vi "Control Panel.vi"(8 "error in (no error)":errorcluster, 11 "Fake CCD in":refnum<class "Synapse CCD.lvclass">) -> (0 "error out":errorcluster, 3 "Fake CCD out":refnum<class "Synapse CCD.lvclass">)   [LabVIEW 2017, in "Synapse CCD.lvclass"]
doc: "(Dynamic) A user-level application that simulates the physical front panel of the Instrument. Provide the user with buttons to manually control features of the instrument, and provide indicators of its current state."
uses:
  Synapse CCD.lvclass
  Areas.ctl
  <vilib>/Utility/error.llb/DialogType.ctl
  Synapse CCD.lvclass/Synapse CCD.ctl
  Spectrometer Triax 550/JY-SPEX-TRIAX/controls.llb/Slits.ctl
  Global/GPIB Numbers.vi
  Spectrometer Triax 550/JY-SPEX-TRIAX/JY-SPEX-TRIAX.lvlib
  Utility Classes/Readable/Readable.lvclass
panel:
  in  "trigger Set CCD warning":bool=TRUE
  out "Changed setting hit Set CCD before continuing":bool
  out "Status":string
  out "Max slit resolution":dbl[unit]
  out "Warning: counts \nwent too high!":bool
  in  "Go to start\nof raster scan":bool
  out "Current snapshot":i32
  out "Number of data \npoints required":i32
  out "JYCCDLib.IJYCCDReqd 1":refnum<k7>
  out "new version of 2D Emma and John Array":i32[][](array[numeric])
  out "where am i?":string
  out "populate fields with member data: CCD private data":T2={"JYCCDLib.IJYCCDReqd"=refnum, "JYMONOLib.IJYMonoReqd"=refnum, "Integration time"=0.01, "ADC"=0, "GAIN"=0, "Areas"=[[1, 1, 1, 1024, 256, 1, 256]], "Most Recent Data Object"=refnum, "Mono Properties"={"Grating"=0, "Center Wavelength"=0.0, "Entrance Slit"=0.0, "Exit Slit"=0.0}, "Coverage"={"Max"=0.0, "Min"=0.0}, "Multi-Acquisitions"={"Dark Subtract?"=FALSE, "Averaging?"=FALSE, "Cosmic Ray Removal?"=FALSE, "# to Average"=0, "Time Between Acq."=0, "Acquisitions Control Array"=[TRUE], "Raw Data"=[], "Processed Data"=[], "Array of Wavelengths"=[]}, "Raster Scan"={"Raster Scan?"=FALSE, "Start"=0.0, "End"=0.0, "Bin width (pixels)"=1, "Bin width (nm)\n(scan resolution)"=3.7e-11, "Number of CCD bins to use each snapshot"=1, "Total possible CCD bins"=20.48, "Warning: counts \nwent too high!"=FALSE}} {"Raster Scan"."Number of CCD bins to use each snapshot" min=1 max=1024 step=1; "Raster Scan"."Bin width (pixels)" min=1 max=1024 step=1; "Mono Properties"."Grating" items=["1200 lines/mm - 500 nm Blaze", "1200 lines/mm - 750 nm Blaze", "600 lines/mm - 1000 nm Blaze"]; "GAIN" items=["High Light", "Best Dynamic", "High Sensitivity"]; "ADC" items=["   20 kHz", "1 MHz", "1 MHz Ultra"]}
  out "Number of snap-\nshots required":i32
  out "Expected time":dbl[unit]
  out "Total possible CCD bins":dbl=20.48
  out "Cosmic Ray Locations":string
  in  "Raster explanation":bool
  in  "image mode":bool
  in  "Repeat pause (ms)":u32
  out "Max value of last snapshot":i32
  in  "Number of CCD bins to use each snapshot":i32=1 min=1 max=1024 step=1
  out "Bin width (nm)\n(scan resolution)":dbl[unit]=3.7e-11
  in  "Bin width (pixels)":i32=1 min=1 max=1024 step=1
  in  "Start":dbl[unit]
  in  "End":dbl[unit]
  in  "Raster Scan":bool
  in  "Repeat Capture":bool
  out "CCD \nInitialized":bool
  out "Spectrometer \nInitialized":bool
  out "Resolution\n(nm/pixel)":dbl[unit] format="%#_3g"
  in  "File Name":path
  in  "Comments":string
  in  "Export\nPlot":bool
  in  "Cosmic Ray\nRemoval?":bool
  out "UnProcessed Spectra":T3(graph)
  in  "# to Average":u32=1
  in  "Averaging?":bool
  in  "Time Between Acq. (ms)":u32
  out "Spectrum":cluster{"Ramp Pattern":dbl[], "X array":dbl[]}[](graph)
  in  "Take Spectrum":bool
  in  "Set CCD":bool
  in  "Set Grating":bool
  in  "stop":bool
  in  "Exit Slit":dbl[unit]
  in  "Entrance Slit":dbl[unit]
  out "Min":dbl[unit]
  out "Max":dbl[unit]
  in  "Center Wavelength":dbl[unit]
  in  "Grating":u16(ring) items=["1200 lines/mm - 500 nm Blaze", "1200 lines/mm - 750 nm Blaze", "600 lines/mm - 1000 nm Blaze"]
  in  "GAIN":u16(ring) caption="Device Name" items=["High Light", "Best Dynamic", "High Sensitivity"]
  in  "ADC":u16(ring) caption="Device Name" items=["   20 kHz", "1 MHz", "1 MHz Ultra"]
  in  "Integration time":dbl[unit]=0.01
  in  "Dark Subtract?":bool
  in  "Copy Actual to Set":bool
  in  "Populate Fields with Member Data":bool
  # "Running this program automatically moves mirror to CCD position"
  # "(unselect to interrupt scan)"
  # "(keep below 65,536 or it saturates)"
  # "Number of CCD bins used in a snapshot must be smaller than Total possible CCD bins"
  # "Debugging stuff"
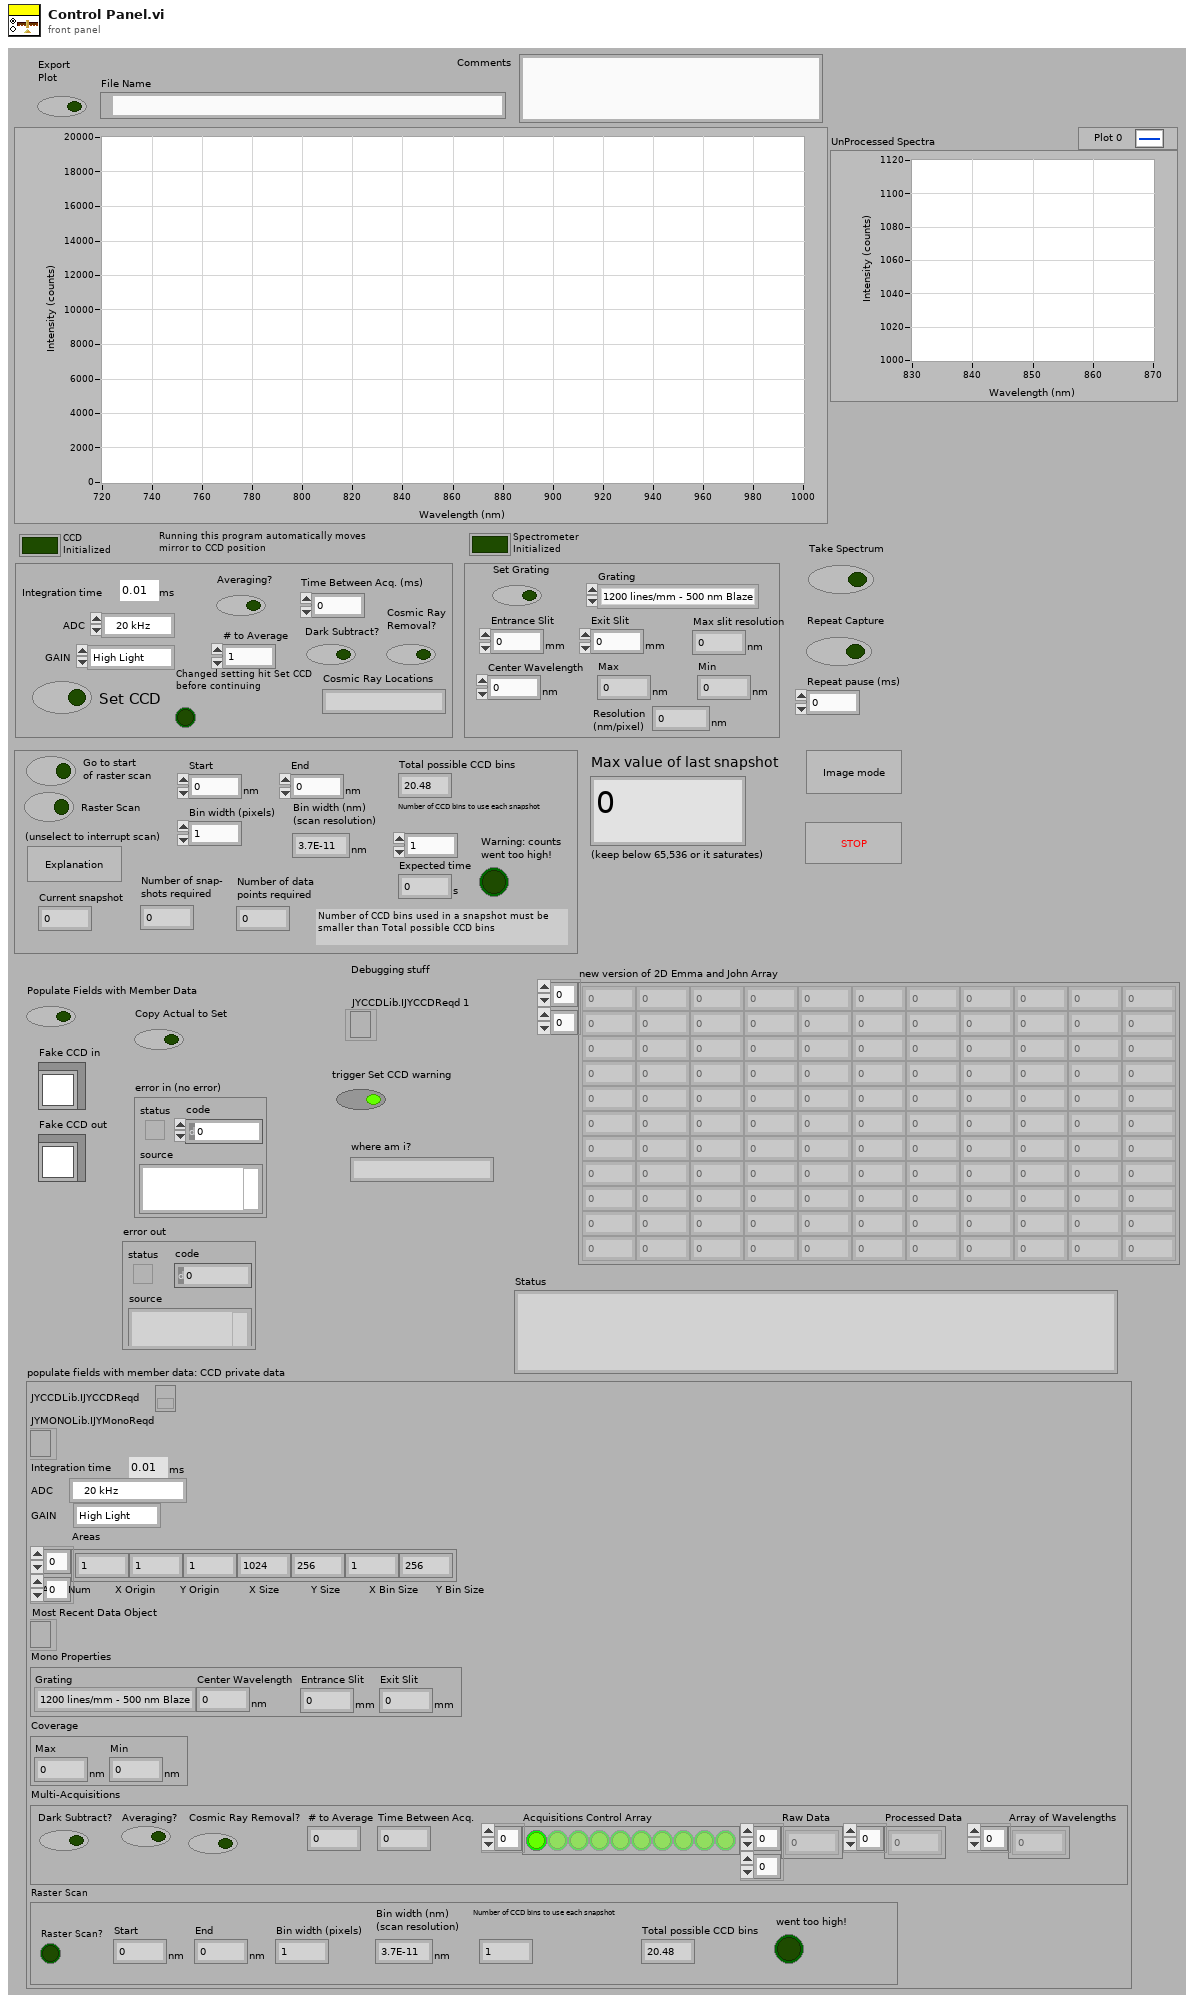
[diagram p1: front panel]
types:
  T1 = typedef "Synapse CCD.lvclass/Areas.ctl" = i32[][]
  T2 = cluster{"JYCCDLib.IJYCCDReqd":refnum<k7>, "JYMONOLib.IJYMonoReqd":refnum<k7>, "Integration time":dbl[unit], "ADC":u16, "GAIN":u16, "Areas":T1, "Most Recent Data Object":refnum<k7>, "Mono Properties":cluster{"Grating":u16, "Center Wavelength":dbl[unit], "Entrance Slit":dbl[unit], "Exit Slit":dbl[unit]}, "Coverage":cluster{"Max":dbl[unit], "Min":dbl[unit]}, "Multi-Acquisitions":cluster{"Dark Subtract?":bool, "Averaging?":bool, "Cosmic Ray Removal?":bool, "# to Average":u32, "Time Between Acq.":u32, "Acquisitions Control Array":bool[], "Raw Data":i32[][], "Processed Data":dbl[], "Array of Wavelengths":dbl[]}, "Raster Scan":cluster{"Raster Scan?":bool, "Start":dbl[unit], "End":dbl[unit], "Bin width (pixels)":i32, "Bin width (nm)\n(scan resolution)":dbl[unit], "Number of CCD bins to use each snapshot":i32, "Total possible CCD bins":dbl, "Warning: counts \nwent too high!":bool}}
  T3 = cluster{"Array of Wavelengths":dbl[], "Raw Data":i32[]}[]
  T4 = typedef "DialogType.ctl" = u16
  T5 = typedef "GPIB Type Def.ctl" = cluster{"Name":string, "bus":dbl, "GPIB":dbl, "GPIB as string":string, "byte":i32, "VISA Resource Name":refnum<visa-resource-name>}
  T6 = typedef "JY-SPEX-TRIAX.lvlib/Slits.ctl" = enum16{"0 (Front/Axial Entrance)", "1 (Side/Lateral Entrance)", "2 (Front/Axial Exit)", "3 (Side/Lateral Exit)"}
  T7 = cluster{"Grating":u16, "Center Wavelength":dbl[unit], "Entrance Slit":dbl[unit], "Exit Slit":dbl[unit]}
  T8 = cluster{"Dark Subtract?":bool, "Averaging?":bool, "Cosmic Ray Removal?":bool, "# to Average":u32, "Time Between Acq.":u32, "Acquisitions Control Array":bool[], "Raw Data":i32[][], "Processed Data":dbl[], "Array of Wavelengths":dbl[]}
  T9 = cluster{"Raster Scan?":bool, "Start":dbl[unit], "End":dbl[unit], "Bin width (pixels)":i32, "Bin width (nm)\n(scan resolution)":dbl[unit], "Number of CCD bins to use each snapshot":i32, "Total possible CCD bins":dbl, "Warning: counts \nwent too high!":bool}
  T10 = cluster{"Array of Wavelengths":dbl[], "Raw Data":i32[]}
  T11 = cluster{"Array of Wavelengths":dbl[], "Processed Data":dbl[]}
  T12 = cluster{"Wavelengths":dbl[], "Avg Counts":dbl[]}[]
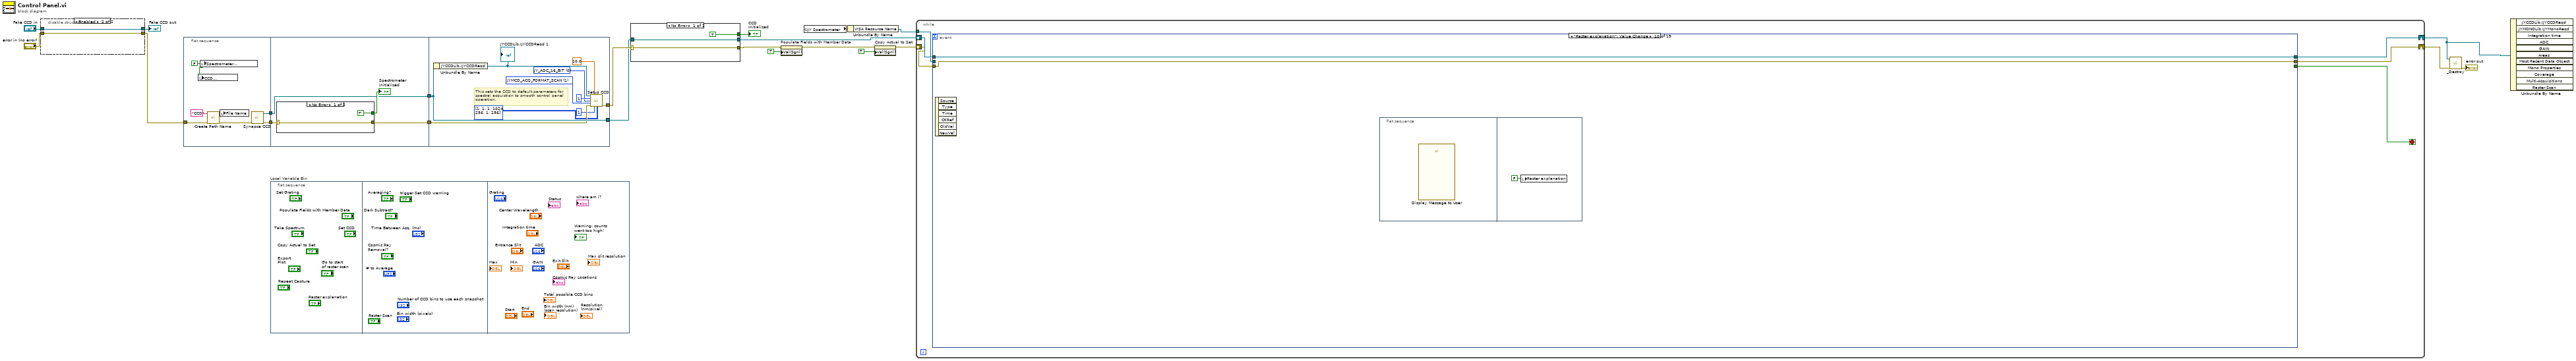
[diagram p0: block diagram]
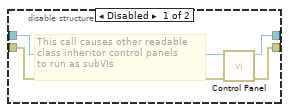
[diagram p2: hidden frame]
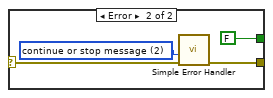
[diagram p3: hidden frame]
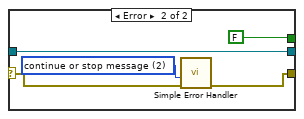
[diagram p4: hidden frame]
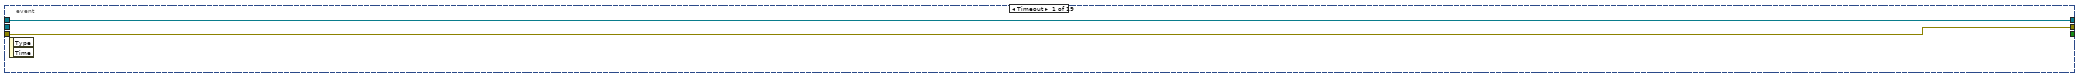
[diagram p5: hidden frame]
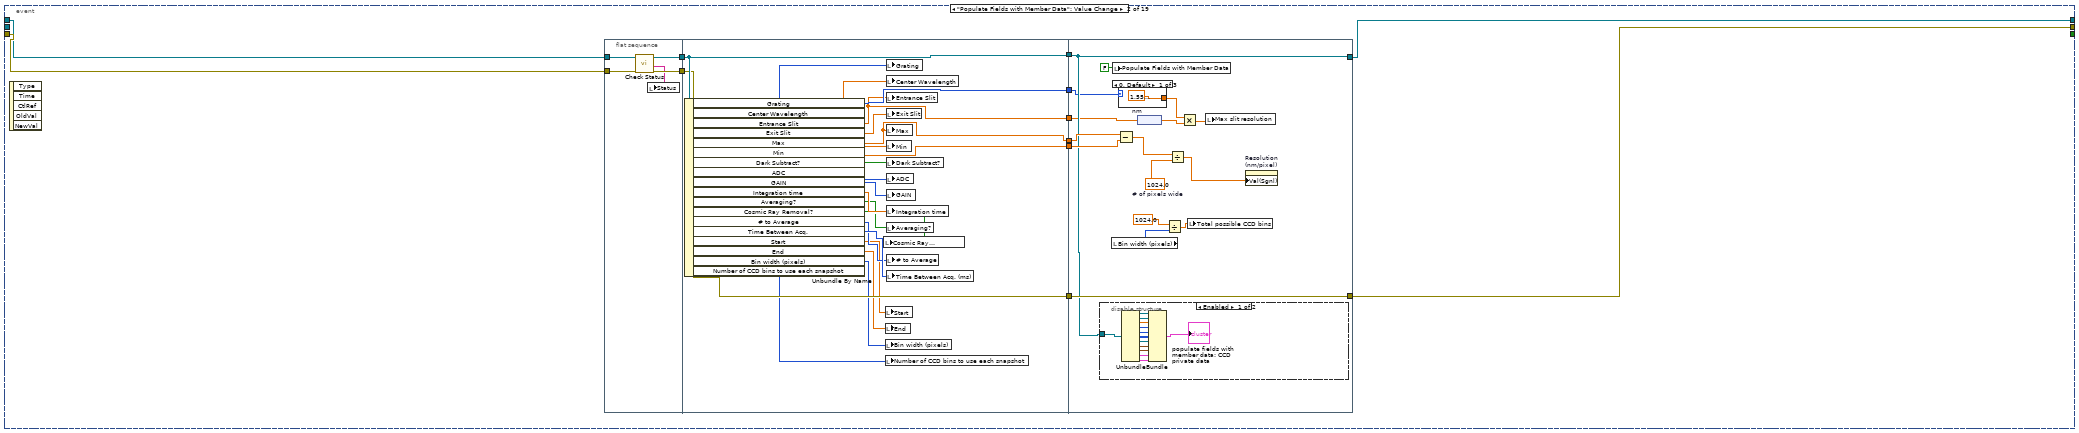
[diagram p6: hidden frame]
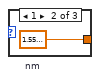
[diagram p7: hidden frame]
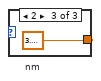
[diagram p8: hidden frame]
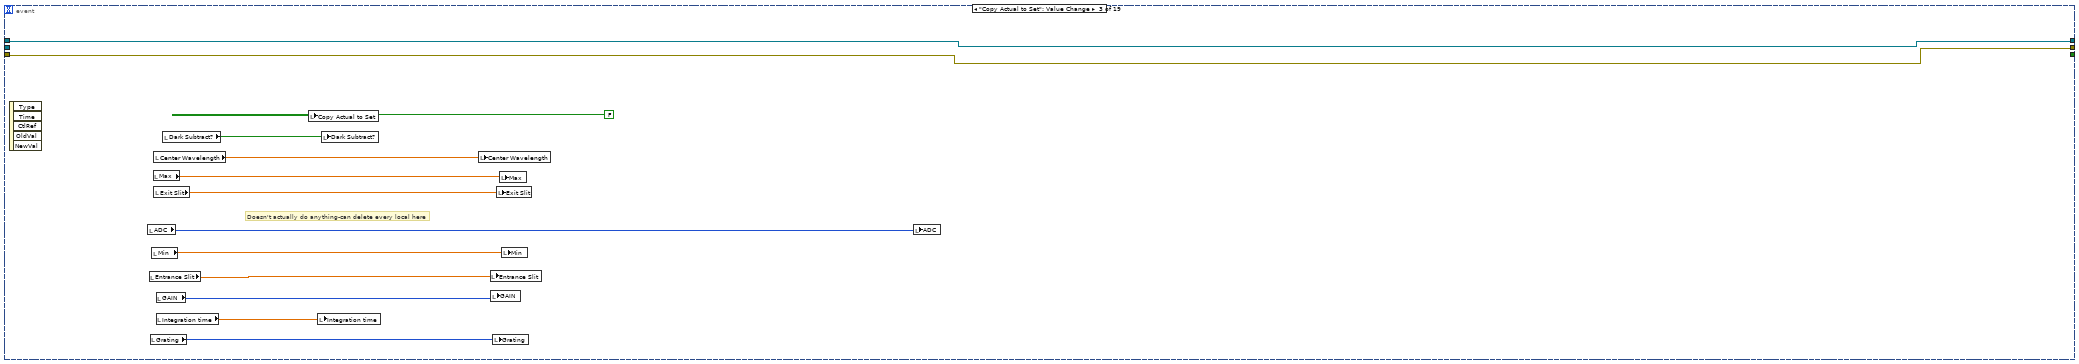
[diagram p10: hidden frame]
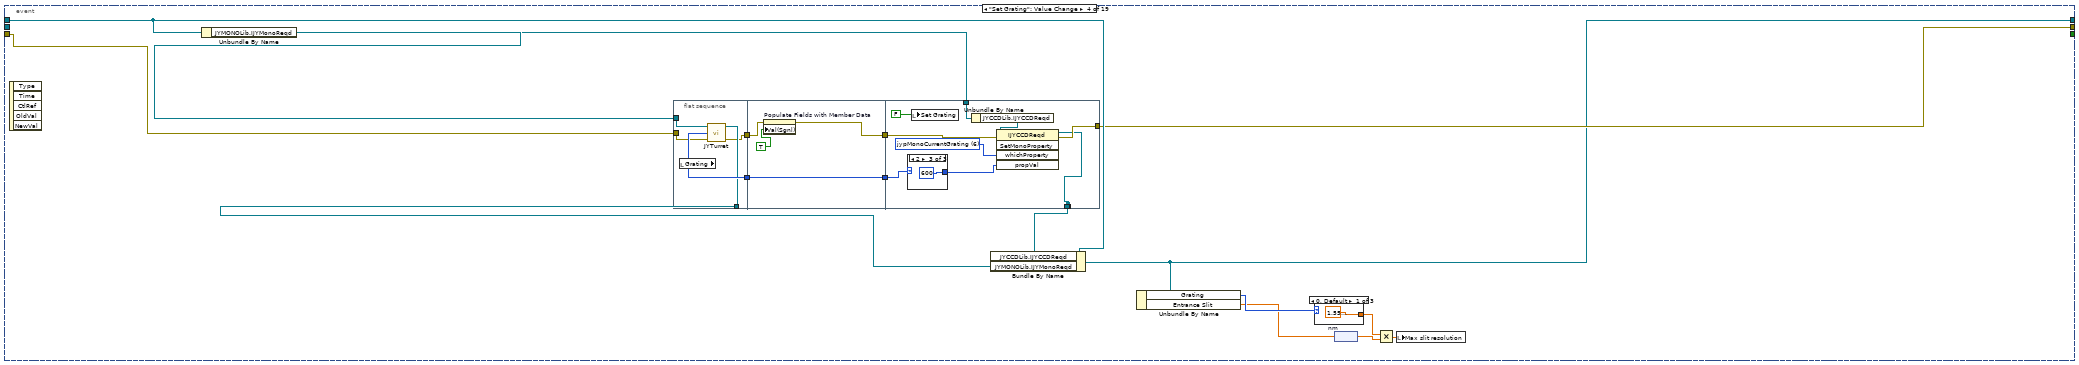
[diagram p11: hidden frame]
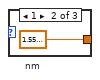
[diagram p12: hidden frame]
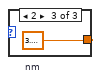
[diagram p13: hidden frame]
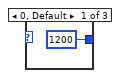
[diagram p14: hidden frame]
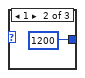
[diagram p15: hidden frame]
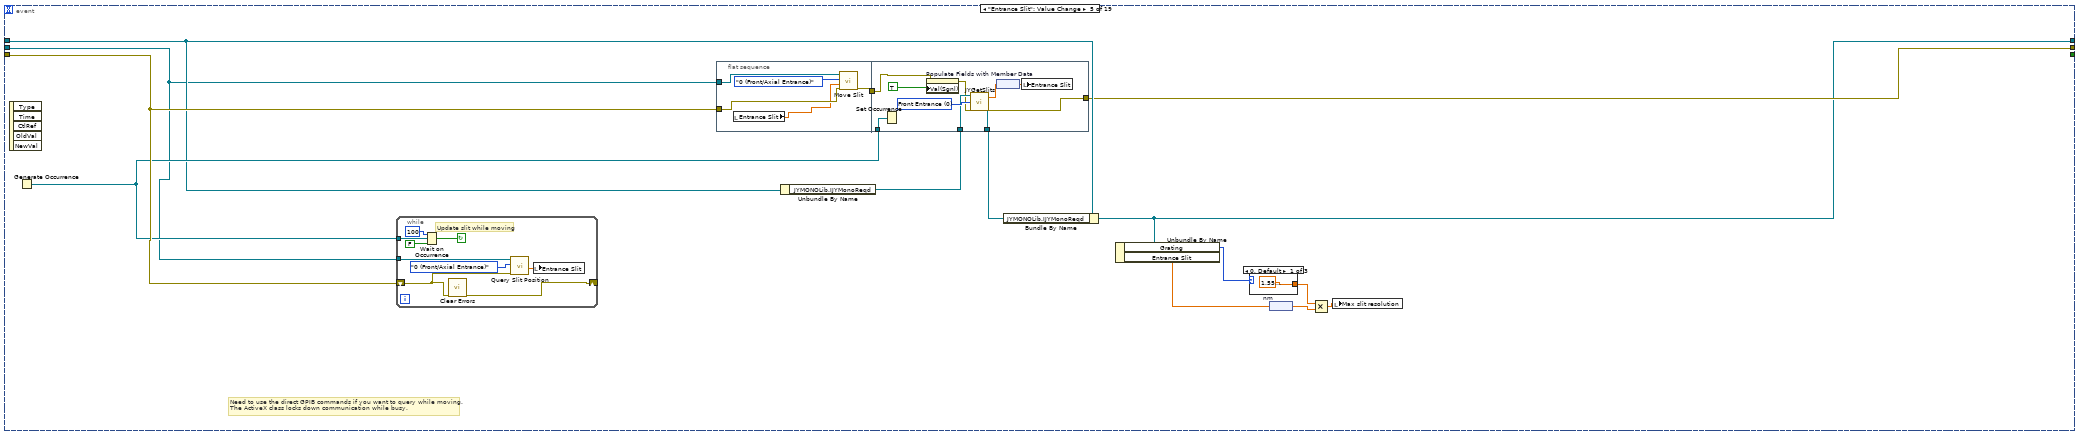
[diagram p16: hidden frame]
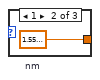
[diagram p17: hidden frame]
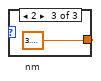
[diagram p18: hidden frame]
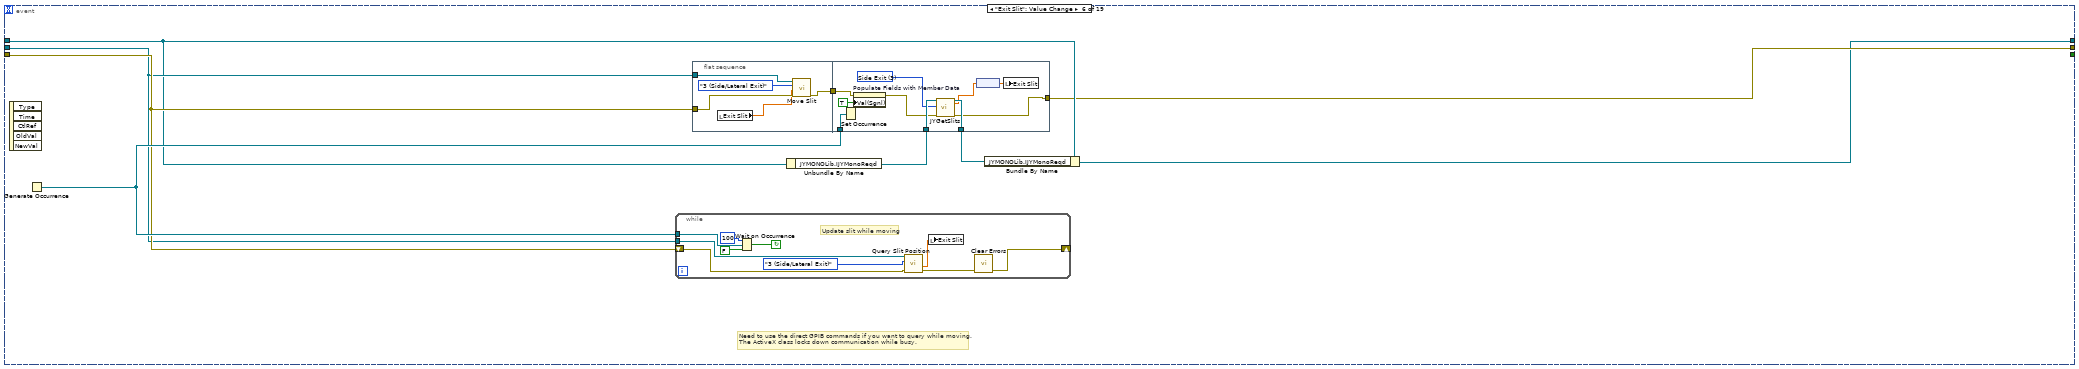
[diagram p19: hidden frame]
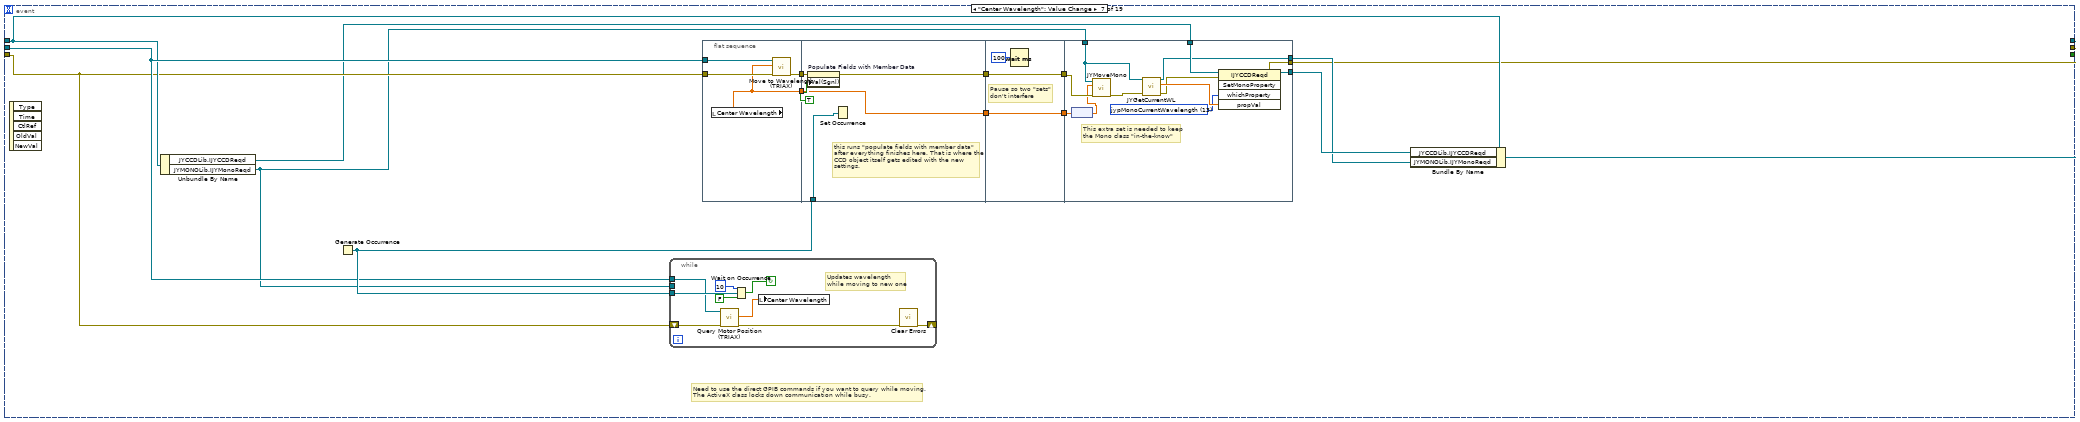
[diagram p20: hidden frame]
diagram:
  n1 = disable-structure shown="Enabled" {
    disable-tunnel: [w26 w28] -> w22
    disable-tunnel: "error in (no error)" -> [w25 w27]
    disable-tunnel: "Fake CCD in" -> [w24 w28]
    disable-tunnel: [w23 w27] -> w19
    frame Disabled {
      # "This call causes other readable\nclass inheritor control panels\nto run as subVIs"
      n2 = call-parent "Control Panel.vi"("error in (no error)"=w25, "Instrument in"=w24) -> ("error out"=w23:errorcluster, "Instrument out"=w26:refnum<class "Synapse CCD.lvclass">)  [unwired: 8 in]
    }
    frame Enabled {
    }
  }
  "Fake CCD out" <- w22
  n3 = flat-sequence {
    tunnel: w19 -> [w33]
    tunnel: [w35] -> w8
    tunnel: [w34] -> w6
    tunnel: w8 -> [w39]
    tunnel: [w38] -> w7
    tunnel: w6 -> [w36]
    tunnel: [w36] -> w5
    tunnel: [w55] -> w2
    tunnel: [w46] -> w13
    tunnel: w7 -> [w49]
    tunnel: w5 -> [w55]
    frame #0 {
      w29 = FALSE ("Spectrometer Initialized")
      n4 = local write "CCD \nInitialized"(w29) -> ()
      n5 = local write "Spectrometer \nInitialized"(w29) -> ()
      n6 = call "Create Path Name.vi"("error in"=w33, "filename"="CCD") -> ("error out"=w32:errorcluster, "path"=w30:path)  [unwired: 1 in, 3 out]
      n7 = local write "File Name"(w30) -> ()
      n8 = call "Synapse CCD.vi"("error in (no error)"=w32) -> ("error out"=w35:errorcluster, "Synapse CCD.lvclass"=w34:refnum<class "Synapse CCD.lvclass">)  [unwired: 9 in]
    }
    frame #1 {
      n9 = case shown="No Error" w39 {
        selector: w39 -> [w41 w44]
        tunnel: [w41 w43] -> w38
        tunnel: [TRUE FALSE] -> w37
        frame No Error {
        }
        frame Error {
          w42 = T4 2 items=["no dialog", "OK message", "continue or stop message", "OK message + warnings", "continue/stop + warnings"] ("type of dialog (OK msg:1)")
          n10 = call <vilib>:"Simple Error Handler.vi"("type of dialog (OK msg:1)"=w42, "error in (no error)"=w44) -> ("error out"=w43:errorcluster)  [unwired: 3 in, 4 out]
        }
      }
      "Spectrometer \nInitialized" <- w37
    }
    frame #2 {
      w50 = 1 items=["JYMCD_ACQ_FORMAT_IMAGE", "JYMCD_ACQ_FORMAT_SCAN"] ("Acquisition type")
      w52 = 0 items=["JY_ADC_16_BIT", "JY_ADC_14_BIT", "JY_ADC_18_BIT"] ("Select ADC")
      # "This sets the CCD to default parameters for\nspectral acquistion to smooth control panel\noperation."
      n11 = Unbundle By Name(w55) -> ("JYCCDLib.IJYCCDReqd"=w54:refnum<k7>)
      "JYCCDLib.IJYCCDReqd 1" <- w54
      n12 = call "Setup CCD.vi"("IJYCCDReqd In"=w54, "Integration time(ms)"=10.0 ("IntegrationTime"), "Select ADC"=w52, "Gain"=1, "Acquisition type"=w50, "error in (no error)"=w49, "numAreas"=1, "areas :"=T1 [[1, 1, 1, 1024, 256, 1, 256]] ("Areas")) -> ("error out"=w46:errorcluster)  [unwired: 5 in, 2 out]
    }
  }
  n13 = flat-sequence "Local Variable Bin" {
    frame #0 {
    }
    frame #1 {
    }
    frame #2 {
    }
  }
  n14 = case shown="No Error" w13 {
    selector: w13 -> [w57 w62]
    tunnel: w2 -> [w58 w63]
    tunnel: [w58 w63] -> w12
    tunnel: [w57 w61] -> w11
    tunnel: [TRUE FALSE] -> w4
    frame No Error {
    }
    frame Error {
      w60 = T4 2 items=["no dialog", "OK message", "continue or stop message", "OK message + warnings", "continue/stop + warnings"] ("type of dialog (OK msg:1)")
      n15 = call <vilib>:"Simple Error Handler.vi"("type of dialog (OK msg:1)"=w60, "error in (no error)"=w62) -> ("error out"=w61:errorcluster)  [unwired: 3 in, 4 out]
    }
  }
  "CCD \nInitialized" <- w4
  n16 = property on="Populate Fields with Member Data" class="Bool (strict)"(error in=w11, "Val(Sgnl)"=TRUE ("Value (Signaling)")) -> (error out=w18:errorcluster)  [unwired: 1 in, 1 out]
  n17 = global read "GPIB Numbers.vi" "JY Spectrometer"() -> (w10:T5)
  n18 = Unbundle By Name(w10) -> ("VISA Resource Name"=w9:refnum<visa-resource-name>)
  n19 = property on="Copy Actual to Set" class="Bool (strict)"(error in=w18, "Val(Sgnl)"=TRUE ("Value (Signaling)")) -> (error out=w17:errorcluster)  [unwired: 1 in, 1 out]
  n20 = while {
    shift-right: [w64] -> w3
    shift-left: w17 -> [w68]
    shift-right: [w65] -> w1
    shift-left: w12 -> [w69]
    tunnel: w9 -> [w67]
    stop <- w66 stop-if-true
    n21 = event shown="[9] \"Raster explanation\": Value Change" {
      selector: _ -> [_ _ _ _ _ _ _ _ _ _ _ _ _ _ _ _ _ _ _]
      dyn-events: _ -> [_ _ _ _ _ _ _ _ _ _ _ _ _ _ _ _ _ _ _]
      timeout: _ -> [_ _ _ _ _ _ _ _ _ _ _ _ _ _ _ _ _ _ _]
      tunnel: w69 -> [w71 w76 w142 w163 w203 w237 w281 w323 w366 w369 w376 w413 w558 w563 w608 w658 _ w724 w741]
      tunnel: w68 -> [w70 w83 w141 w165 w206 w241 w273 w331 w365 w368 w377 w414 w557 w564 w609 w661 _ w723 w742]
      tunnel: [w70 w74 w141 w160 w200 w236 w272 w322 w365 w368 w371 w409 w557 w564 w609 w653 _ w721 w742] -> w64
      tunnel: [w71 w75 w142 w157 w197 w235 w271 w321 w366 w369 w380 w410 w558 w562 w607 w659 _ w722 w741] -> w65
      tunnel: [_ _ _ _ _ _ _ _ _ _ _ _ _ _ _ _ _ _ "stop"] -> w66
      tunnel: w67 -> [_ _ _ _ w202 w239 w282 _ _ _ _ w412 _ _ _ _ _ _ _]
      event Timeout {
        n22 = event-data() -> ()  [unwired: 1 in, 2 out]
      }
      event "Populate Fields with Member Data": Value Change {
        n23 = event-data() -> ()  [unwired: 1 in, 5 out]
        n24 = flat-sequence {
          tunnel: w83 -> [w86]
          tunnel: w76 -> [w88]
          tunnel: [w87] -> w80
          tunnel: [w85] -> w79
          tunnel: [w102] -> w82
          tunnel: [w95] -> w81
          tunnel: w80 -> [w102]
          tunnel: w79 -> [w95]
          tunnel: [w97] -> w78
          tunnel: [w96] -> w77
          tunnel: [w94] -> w73
          tunnel: [w93] -> w72
          tunnel: [w124] -> w74
          tunnel: [w115] -> w75
          tunnel: w82 -> [w115]
          tunnel: w81 -> [w124]
          tunnel: w78 -> [w119]
          tunnel: w77 -> [w120]
          tunnel: w73 -> [w113]
          tunnel: w72 -> [w110]
          frame #0 {
            n25 = call-dynamic "Check Status.vi"("error in (no error)"=w86, "Synapse CCD in"=w88) -> ("error out"=w85:errorcluster, "Status"=w84:string, "Synapse CCD out"=w87:refnum<class "Synapse CCD.lvclass">)  [unwired: 6 in, 1 out]
            n26 = local write "Status"(w84) -> ()
          }
          frame #1 {
            n27 = Unbundle By Name(w102) -> ("Grating"=w94:u16, "Center Wavelength"=w108:dbl[unit], "Entrance Slit"=w93:dbl[unit], "Exit Slit"=w107:dbl[unit], "Max"=w97:dbl[unit], "Min"=w96:dbl[unit], "Dark Subtract?"=w106:bool, "ADC"=w105:u16, "GAIN"=w104:u16, "Integration time"=w103:dbl[unit], "Averaging?"=w98:bool, "Cosmic Ray Removal?"=w99:bool, "# to Average"=w100:u32, "Time Between Acq."=w101:u32, "Start"=w92:dbl[unit], "End"=w91:dbl[unit], "Bin width (pixels)"=w90:i32, "Number of CCD bins to use each snapshot"=w89:i32)
            n28 = local write "Cosmic Ray\nRemoval?"(w99) -> ()
            n29 = local write "Start"(w92) -> ()
            n30 = local write "End"(w91) -> ()
            n31 = local write "Bin width (pixels)"(w90) -> ()
            n32 = local write "Number of CCD bins to use each snapshot"(w89) -> ()
            n33 = local write "Grating"(w94) -> ()
            n34 = local write "Center Wavelength"(w108) -> ()
            n35 = local write "Entrance Slit"(w93) -> ()
            n36 = local write "Exit Slit"(w107) -> ()
            n37 = local write "Max"(w97) -> ()
            n38 = local write "Min"(w96) -> ()
            n39 = local write "Dark Subtract?"(w106) -> ()
            n40 = local write "ADC"(w105) -> ()
            n41 = local write "GAIN"(w104) -> ()
            n42 = local write "Integration time"(w103) -> ()
            n43 = local write "Averaging?"(w98) -> ()
            n44 = local write "# to Average"(w100) -> ()
            n45 = local write "Time Between Acq. (ms)"(w101) -> ()
          }
          frame #2 {
            w121 = 1024.0  # # of pixels wide
            n46 = disable-structure shown="Enabled" {
              disable-tunnel: w115 -> [w132 _]
              frame Enabled {
                n47 = Unbundle(w132) -> (w140:refnum<k7>, w139:refnum<k7>, w138:dbl[unit], w137:u16, w136:u16, w135:T1, w134:refnum<k7>, w133:T7, w131:cluster{"Max":dbl[unit], "Min":dbl[unit]}, w130:T8, w129:T9)
                n48 = Bundle("JYCCDLib.IJYCCDReqd"=w140, "JYMONOLib.IJYMonoReqd"=w139, "Integration time"=w138, "ADC"=w137, "GAIN"=w136, "Areas"=w135, "Most Recent Data Object"=w134, "Mono Properties"=w133, "Coverage"=w131, "Multi-Acquisitions"=w130, "Raster Scan"=w129) -> (→"populate fields with member data: CCD private data":T2)  [unwired: 1 in]
              }
              frame Disabled {
              }
            }
            n49 = local read "Bin width (pixels)"() -> (w117:i32)
            n50 = local write "Populate Fields with Member Data"(FALSE ("Populate Fields with Member Data")) -> ()
            n51 = Subtract(x=w119, y=w120) -> (x-y=w122:dbl[unit])
            n52 = case shown="0, Default" w113 {
              tunnel: [w125 w126 w127] -> w112
              frame 0, Default {
                w125 = dbl[unit] 1.5500000000000002e-09  # nm
              }
              frame 1 {
                w126 = dbl[unit] 1.5500000000000002e-09  # nm
              }
              frame 2 {
                w127 = dbl[unit] 3.1000000000000005e-09  # nm
              }
            }
            n53 = node(w110) -> (w109:dbl)
            n54 = Divide(x=1024.0, y=w117) -> (x/y=w118:dbl)
            n55 = Divide(x=w122, y=w121) -> (x/y=w114:dbl[unit])
            n56 = Multiply(x=w112, y=w109) -> (x*y=w111:dbl[unit])
            n57 = local write "Total possible CCD bins"(w118) -> ()
            n58 = local write "Max slit resolution"(w111) -> ()
            n59 = property on="Resolution\n(nm/pixel)" class="DigNum (strict)"("Val(Sgnl)"=w114) -> ()  [unwired: 2 in, 2 out]
          }
        }
      }
      event "Copy Actual to Set": Value Change {
        # "Doesn't actually do anything-can delete every local here"
        n60 = event-data() -> ()  [unwired: 1 in, 5 out]
        n61 = local read "ADC"() -> (w153:u16)
        n62 = local read "Entrance Slit"() -> (w149:dbl[unit])
        n63 = local read "Grating"() -> (w146:u16)
        n64 = local read "Min"() -> (w150:dbl[unit])
        n65 = local read "Max"() -> (w144:dbl[unit])
        n66 = local read "Center Wavelength"() -> (w152:dbl[unit])
        n67 = local read "Exit Slit"() -> (w148:dbl[unit])
        n68 = local read "GAIN"() -> (w147:u16)
        n69 = local read "Integration time"() -> (w145:dbl[unit])
        n70 = local read "Dark Subtract?"() -> (w151:bool)
        n71 = local write "Copy Actual to Set"(FALSE ("Copy Actual to Set")) -> ()
        n72 = local write "Integration time"(w145) -> ()
        n73 = local write "Dark Subtract?"(w151) -> ()
        n74 = local write "Center Wavelength"(w152) -> ()
        n75 = local write "Entrance Slit"(w149) -> ()
        n76 = local write "GAIN"(w147) -> ()
        n77 = local write "Grating"(w146) -> ()
        n78 = local write "Exit Slit"(w148) -> ()
        n79 = local write "Max"(w144) -> ()
        n80 = local write "Min"(w150) -> ()
        n81 = local write "ADC"(w153) -> ()
      }
      event "Set Grating": Value Change {
        n82 = event-data() -> ()  [unwired: 1 in, 5 out]
        n83 = Unbundle By Name(w163) -> ("JYMONOLib.IJYMonoReqd"=w164:refnum<k7>)
        n84 = flat-sequence {
          tunnel: w164 -> [w175]
          tunnel: w165 -> [w176]
          tunnel: [w173] -> w169
          tunnel: [w177] -> w167
          tunnel: [w174] -> w162
          tunnel: w169 -> [w181]
          tunnel: [w180] -> w168
          tunnel: w167 -> [w180]
          tunnel: [w178] -> w166
          tunnel: [w183] -> w160
          tunnel: w168 -> [w189]
          tunnel: w166 -> [w186]
          tunnel: [w182] -> _
          tunnel: w163 -> [w188]
          tunnel: [w182] -> w161
          frame #0 {
            n85 = local read "Grating"() -> (w177:u16)
            n86 = call "JYTurret.vi"("error in (no error)"=w176, "Grating Index"=w177, "JYMONOLib.IJYMonoReqd In"=w175) -> ("error out"=w173:errorcluster, "JYMONOLib.IJYMonoReqd Out"=w174:refnum<k7>)  [unwired: 1 out]
          }
          frame #1 {
            n87 = property on="Populate Fields with Member Data" class="Bool (strict)"(error in=w181, "Val(Sgnl)"=TRUE ("Value (Signaling)")) -> (error out=w178:errorcluster)  [unwired: 1 in, 1 out]
          }
          frame #2 {
            w187 = 6 items=["jyUndefined", "jypMonoLinearDispersion", "jypMonoBacklashAmount", "jypMonoStepsPerUnit", "jypMonoBaseUnits", "jypMonoBaseGrating", "jypMonoCurrentGrating", "jypMonoMaxLimit", "jypMonoMinLimit", "jypMonoTiltAngle", "jypMonoIncludedAngle", "jypMonoFocalLength", "jypMonoOrder", "jypMonoCurrentWavelength", "jypMonoMCDWavelengthDirection", "jypBandpassUnits", "jypSlitMaxLimit", "jypSlitMinLimit", "jypSlitBackLashAmount", "jypSlitBaseUnits", "jypSlitStepsPerUnit", "jypLaserLine", "jypTotalHardwarePropertiesPlusOne", "jypCurrentTurretPosition"] ("whichProperty")
            n88 = case shown="2" w189 {
              tunnel: [u16 1200 u16 1200 u16 600] -> w184
              frame 0, Default {
              }
              frame 1 {
              }
              frame 2 {
              }
            }
            n89 = local write "Set Grating"(FALSE ("Set Spectrometer")) -> ()
            n90 = Unbundle By Name(w188) -> ("JYCCDLib.IJYCCDReqd"=w185:refnum<k7>)
            n91 = invoke class="IJYCCDReqd" method="SetMonoProperty"(reference=w185, error in=w186, "whichProperty"=w187, "propVal"=w184) -> (reference out=w182:refnum<k7>, error out=w183:errorcluster)  [unwired: 1 in, 3 out]
          }
        }
        n92 = Bundle By Name(cluster=w163, "JYCCDLib.IJYCCDReqd"=w161, "JYMONOLib.IJYMonoReqd"=w162) -> (w157:refnum<class "Synapse CCD.lvclass">)
        n93 = Unbundle By Name(w157) -> ("Grating"=w156:u16, "Entrance Slit"=w155:dbl[unit])
        n94 = case shown="0, Default" w156 {
          tunnel: [w170 w171 w172] -> w159
          frame 0, Default {
            w170 = dbl[unit] 1.5500000000000002e-09  # nm
          }
          frame 1 {
            w171 = dbl[unit] 1.5500000000000002e-09  # nm
          }
          frame 2 {
            w172 = dbl[unit] 3.1000000000000005e-09  # nm
          }
        }
        n95 = node(w155) -> (w158:dbl)
        n96 = Multiply(x=w159, y=w158) -> (x*y=w154:dbl[unit])
        n97 = local write "Max slit resolution"(w154) -> ()
      }
      event "Entrance Slit": Value Change {
        # "Need to use the direct GPIB commands if you want to query while moving.\nThe ActiveX class locks down communication while busy."
        n98 = event-data() -> ()  [unwired: 1 in, 5 out]
        n99 = Generate Occurrence() -> (w205:refnum<k4>)
        n100 = while {
          tunnel: w205 -> [w219]
          shift-right: [w211] -> _
          shift-left: w206 -> [w212]
          tunnel: w202 -> [w215]
          stop <- w218 continue-if-true
          # "Update slit while moving"
          n101 = Wait on Occurrence(1:FALSE ("ignore previous (T)"), 2:w219, 3:100 ("ms timeout (-1)")) -> (0:w218:bool)
          n102 = call <vilib>:"Clear Errors.vi"("error in (no error)"=w212) -> ("error out"=w211:errorcluster)  [unwired: 5 in, 1 out]
          n103 = call "Query Slit Position.vi"("error in (no error)"=w212, "Slit (Front/Axial Entrance)"=Slits."0 (Front/Axial Entrance)", "VISA resource name"=w215) -> ("Slit Position"=w213:dbl[unit])  [unwired: 6 in, 2 out]
          n104 = local write "Entrance Slit"(w213) -> ()
        }
        n105 = flat-sequence {
          tunnel: w206 -> [w221]
          tunnel: [w224] -> w207
          tunnel: w202 -> [w222]
          tunnel: w207 -> [w229]
          tunnel: [w225] -> w200
          tunnel: w205 -> [w234]
          tunnel: w204 -> [w232]
          tunnel: [w230] -> w201
          frame #0 {
            n106 = local read "Entrance Slit"() -> (w220:dbl[unit])
            n107 = call "Move Slit.vi"("error in (no error)"=w221, "Desired Slit Position"=w220, "Slit (Front/Axial Entrance)"=Slits."0 (Front/Axial Entrance)", "VISA resource name"=w222) -> ("error out"=w224:errorcluster)  [unwired: 6 in, 1 out]
          }
          frame #1 {
            w233 = u16 0 items=["Front Entrance", "Side Entrance", "Front Exit", "Side Exit", "First Intermediate", "Second Intermediate"] ("Slit")
            n108 = Set Occurrence(w234) -> ()
            n109 = property on="Populate Fields with Member Data" class="Bool (strict)"(error in=w229, "Val(Sgnl)"=TRUE ("Value (Signaling)")) -> (error out=w227:errorcluster)  [unwired: 1 in, 1 out]
            n110 = call "JYGetSlits.vi"("MonoRefNum IN"=w232, "Slit"=w233, "error in (no error)"=w227) -> ("MonoRefNum Out"=w230:refnum<k7>, "Slit Width"=w226:dbl, "error out"=w225:errorcluster)  [unwired: 13 in, 1 out]
            n111 = node(w226) -> (w231:dbl[unit])
            n112 = local write "Entrance Slit"(w231) -> ()
          }
        }
        n113 = Unbundle By Name(w203) -> ("JYMONOLib.IJYMonoReqd"=w204:refnum<k7>)
        n114 = Bundle By Name(cluster=w203, "JYMONOLib.IJYMonoReqd"=w201) -> (w197:refnum<class "Synapse CCD.lvclass">)
        n115 = Unbundle By Name(w197) -> ("Grating"=w196:u16, "Entrance Slit"=w195:dbl[unit])
        n116 = case shown="0, Default" w196 {
          tunnel: [w208 w209 w210] -> w199
          frame 0, Default {
            w208 = dbl[unit] 1.5500000000000002e-09  # nm
          }
          frame 1 {
            w209 = dbl[unit] 1.5500000000000002e-09  # nm
          }
          frame 2 {
            w210 = dbl[unit] 3.1000000000000005e-09  # nm
          }
        }
        n117 = node(w195) -> (w198:dbl)
        n118 = Multiply(x=w199, y=w198) -> (x*y=w194:dbl[unit])
        n119 = local write "Max slit resolution"(w194) -> ()
      }
      event "Exit Slit": Value Change {
        # "Need to use the direct GPIB commands if you want to query while moving.\nThe ActiveX class locks down communication while busy."
        n120 = event-data() -> ()  [unwired: 1 in, 5 out]
        n121 = Generate Occurrence() -> (w242:refnum<k4>)
        n122 = while {
          tunnel: w242 -> [w253]
          shift-right: [w244] -> _
          shift-left: w241 -> [w248]
          tunnel: w239 -> [w247]
          stop <- w251 continue-if-true
          # "Update slit while moving"
          n123 = Wait on Occurrence(1:FALSE ("ignore previous (T)"), 2:w253, 3:100 ("ms timeout (-1)")) -> (0:w251:bool)
          n124 = call "Query Slit Position.vi"("error in (no error)"=w248, "Slit (Front/Axial Entrance)"=Slits."3 (Side/Lateral Exit)", "VISA resource name"=w247) -> ("error out"=w245:errorcluster, "Slit Position"=w249:dbl[unit])  [unwired: 6 in, 1 out]
          n125 = local write "Exit Slit"(w249) -> ()
          n126 = call <vilib>:"Clear Errors.vi"("error in (no error)"=w245) -> ("error out"=w244:errorcluster)  [unwired: 5 in, 1 out]
        }
        n127 = flat-sequence {
          tunnel: w241 -> [w257]
          tunnel: [w254] -> w243
          tunnel: w239 -> [w256]
          tunnel: w243 -> [w262]
          tunnel: [w259] -> w236
          tunnel: w242 -> [w267]
          tunnel: w240 -> [w266]
          tunnel: [w263] -> w238
          frame #0 {
            n128 = local read "Exit Slit"() -> (w255:dbl[unit])
            n129 = call "Move Slit.vi"("error in (no error)"=w257, "Desired Slit Position"=w255, "Slit (Front/Axial Entrance)"=Slits."3 (Side/Lateral Exit)", "VISA resource name"=w256) -> ("error out"=w254:errorcluster)  [unwired: 6 in, 1 out]
          }
          frame #1 {
            w265 = u16 3 items=["Front Entrance", "Side Entrance", "Front Exit", "Side Exit", "First Intermediate", "Second Intermediate"] ("Slit")
            n130 = Set Occurrence(w267) -> ()
            n131 = property on="Populate Fields with Member Data" class="Bool (strict)"(error in=w262, "Val(Sgnl)"=TRUE ("Value (Signaling)")) -> (error out=w261:errorcluster)  [unwired: 1 in, 1 out]
            n132 = call "JYGetSlits.vi"("MonoRefNum IN"=w266, "Slit"=w265, "error in (no error)"=w261) -> ("MonoRefNum Out"=w263:refnum<k7>, "Slit Width"=w260:dbl, "error out"=w259:errorcluster)  [unwired: 13 in, 1 out]
            n133 = node(w260) -> (w264:dbl[unit])
            n134 = local write "Exit Slit"(w264) -> ()
          }
        }
        n135 = Unbundle By Name(w237) -> ("JYMONOLib.IJYMonoReqd"=w240:refnum<k7>)
        n136 = Bundle By Name(cluster=w237, "JYMONOLib.IJYMonoReqd"=w238) -> (w235:refnum<class "Synapse CCD.lvclass">)
      }
      event "Center Wavelength": Value Change {
        # "Need to use the direct GPIB commands if you want to query while moving.\nThe ActiveX class locks down communication while busy."
        n137 = event-data() -> ()  [unwired: 1 in, 5 out]
        n138 = Unbundle By Name(w281) -> ("JYCCDLib.IJYCCDReqd"=w270:refnum<k7>, "JYMONOLib.IJYMonoReqd"=w269:refnum<k7>)
        n139 = Generate Occurrence() -> (w283:refnum<k4>)
        n140 = while {
          tunnel: w283 -> [w293]
          tunnel: w269 -> [_]
          shift-right: [w289] -> _
          shift-left: w273 -> [w288]
          tunnel: w282 -> [w285]
          stop <- w291 continue-if-true
          # "Updates wavelength\nwhile moving to new one"
          n141 = call "Query Motor Position (TRIAX).vi"("error in (no error)"=w288, "VISA resource name"=w285) -> ("error out"=w287:errorcluster, "wavelength"=w286:dbl[unit])  [unwired: 7 in, 1 out]
          n142 = Wait on Occurrence(1:FALSE ("ignore previous (T)"), 2:w293, 3:10 ("ms timeout (-1)")) -> (0:w291:bool)
          n143 = local write "Center Wavelength"(w286) -> ()
          n144 = call <vilib>:"Clear Errors.vi"("error in (no error)"=w287) -> ("error out"=w289:errorcluster)  [unwired: 5 in, 1 out]
        }
        n145 = flat-sequence {
          tunnel: w273 -> [w297]
          tunnel: [w296] -> w284
          tunnel: w282 -> [w295]
          tunnel: [w294] -> w278
          tunnel: w284 -> [w301]
          tunnel: [w300] -> w277
          tunnel: w283 -> [w298]
          tunnel: [w299] -> w275
          tunnel: w278 -> [w299]
          tunnel: w277 -> [w305]
          tunnel: [w305] -> w276
          tunnel: w275 -> [w304]
          tunnel: [w304] -> w274
          tunnel: [w317] -> w272
          tunnel: w276 -> [w310]
          tunnel: w270 -> [w316]
          tunnel: [w313] -> w280
          tunnel: [w307] -> w279
          tunnel: w274 -> [w311]
          tunnel: w269 -> [w306]
          frame #0 {
            n146 = local read "Center Wavelength"() -> (w294:dbl[unit])
            n147 = call "Move to Wavelength (TRIAX).vi"("error in (no error)"=w297, "Target wavelength"=w294, "VISA resource name"=w295) -> ("error out"=w296:errorcluster)  [unwired: 7 in, 1 out]
          }
          frame #1 {
            # "this runs \"populate fields with member data\" \nafter everything finishes here. That is where the \nCCD object itself gets edited with the new \nsettings."
            n148 = property on="Populate Fields with Member Data" class="Bool (strict)"(error in=w301, "Val(Sgnl)"=TRUE ("Value (Signaling)")) -> (error out=w300:errorcluster)  [unwired: 1 in, 1 out]
            n149 = Set Occurrence(w298) -> ()
          }
          frame #2 {
            # "Pause so two \"sets\" \ndon't interfere"
            n150 = Wait (ms)(milliseconds to wait=u32 100) -> ()  [unwired: 1 out]
          }
          frame #3 {
            w308 = 13 items=["jyUndefined", "jypMonoLinearDispersion", "jypMonoBacklashAmount", "jypMonoStepsPerUnit", "jypMonoBaseUnits", "jypMonoBaseGrating", "jypMonoCurrentGrating", "jypMonoMaxLimit", "jypMonoMinLimit", "jypMonoTiltAngle", "jypMonoIncludedAngle", "jypMonoFocalLength", "jypMonoOrder", "jypMonoCurrentWavelength", "jypMonoMCDWavelengthDirection", "jypBandpassUnits", "jypSlitMaxLimit", "jypSlitMinLimit", "jypSlitBackLashAmount", "jypSlitBaseUnits", "jypSlitStepsPerUnit", "jypLaserLine", "jypTotalHardwarePropertiesPlusOne", "jypCurrentTurretPosition"] ("whichProperty")
            # "This extra set is needed to keep \nthe Mono class \"in-the-know\""
            n151 = node(w311) -> (w309:dbl)
            n152 = call "JYMoveMono.vi"("error in (no error)"=w310, 10:w309, "JYMONOLib.IJYMonoReqd"=w306) -> ("error out"=w312:errorcluster)  [unwired: 8 in]
            n153 = call "JYGetCurrentWL.vi"("error in (no error)"=w312, "JYMONOLib.IJYMonoReqd In"=w306) -> ("error out"=w314:errorcluster, "Current WL"=w315:dbl, "JYMONOLib.IJYMonoReqd Out"=w307:refnum<k7>)  [unwired: 6 in, 1 out]
            n154 = invoke class="IJYCCDReqd" method="SetMonoProperty"(reference=w316, error in=w314, "whichProperty"=w308, "propVal"=w315) -> (reference out=w313:refnum<k7>, error out=w317:errorcluster)  [unwired: 1 in, 3 out]
          }
        }
        n155 = Bundle By Name(cluster=w281, "JYCCDLib.IJYCCDReqd"=w280, "JYMONOLib.IJYMonoReqd"=w279) -> (w271:refnum<class "Synapse CCD.lvclass">)
      }
      event "Set CCD": Value Change {
        # "ADC Query Method is broken\n\nKeep track of it manually in \nmember data"
        n156 = event-data() -> ()  [unwired: 1 in, 5 out]
        n157 = Unbundle By Name(w323) -> ("JYCCDLib.IJYCCDReqd"=w318:refnum<k7>, "Areas"=w326:T1)
        n158 = local write "where am i?"("step1" ("where am i?")) -> ()
        n159 = Index Array(array=w326, index (col)=0 ("index (row)")) -> (element=w325:i32[])  [unwired: 1 in]
        n160 = Array Size(array=w325) -> (size(s)=w324:i32)
        n161 = flat-sequence {
          tunnel: w324 -> [w345]
          tunnel: w326 -> [w344]
          tunnel: w318 -> [w338]
          tunnel: w331 -> [w339]
          tunnel: [w342] -> w330
          tunnel: w323 -> [w341]
          tunnel: [w333] -> w327
          tunnel: w330 -> [w351]
          tunnel: [w351] -> w328
          tunnel: [w347] -> w321
          tunnel: w327 -> [w350]
          tunnel: w328 -> [w358]
          tunnel: [w357] -> w320
          tunnel: [w363] -> w322
          tunnel: w320 -> [w363]
          frame #0 {
            w336 = 1 items=["JYMCD_ACQ_FORMAT_IMAGE", "JYMCD_ACQ_FORMAT_SCAN"] ("Acquisition type")
            n162 = local read "Integration time"() -> (w343:dbl[unit])
            n163 = node(w343) -> (w335:dbl)
            n164 = local read "GAIN"() -> (w337:u16)
            n165 = local read "ADC"() -> (w334:u16)
            n166 = call "Setup CCD.vi"("IJYCCDReqd In"=w338, "Integration time(ms)"=w335, "Select ADC"=w334, "Gain"=w337, "Acquisition type"=w336, "error in (no error)"=w339, "numAreas"=w345, "areas :"=w344) -> ("IJYCCDReqd Out"=w340:refnum<k7>, "error out"=w342:errorcluster)  [unwired: 5 in, 1 out]
            n167 = local write "where am i?"("step2" ("where am i?")) -> ()
            n168 = Bundle By Name(cluster=w341, "ADC"=w334, "JYCCDLib.IJYCCDReqd"=w340) -> (w333:refnum<class "Synapse CCD.lvclass">)
          }
          frame #1 {
            n169 = local read "Time Between Acq. (ms)"() -> (w352:u32)
            n170 = local read "Averaging?"() -> (w349:bool)
            n171 = local read "Cosmic Ray\nRemoval?"() -> (w348:bool)
            n172 = local read "Dark Subtract?"() -> (w354:bool)
            n173 = local read "# to Average"() -> (w353:u32)
            n174 = local write "where am i?"("step3" ("where am i?")) -> ()
            n175 = call "Setup Multi Acq.vi"("# of Scans"=w353, "Time Between Acq (ms)"=w352, "Cosmic Ray Removal?"=w348, "Averaging?"=w349, "Dark Subtract?"=w354, "Synapse CCD.lvclass In"=w350) -> ("Synapse CCD.lvclass Out"=w347:refnum<class "Synapse CCD.lvclass">)  [unwired: 5 in]
          }
          frame #2 {
            n176 = property on="Populate Fields with Member Data" class="Bool (strict)"(error in=w358, "Val(Sgnl)"=TRUE) -> (error out=w357:errorcluster)  [unwired: 1 in, 1 out]
            n177 = local write "where am i?"("step4" ("where am i?")) -> ()
            n178 = Wait (ms)(milliseconds to wait=u32 100) -> ()  [unwired: 1 out]
          }
          frame #3 {
            n179 = local write "where am i?"("step5" ("where am i?")) -> ()
            n180 = local write "Set CCD"(FALSE ("Set CCD")) -> ()
            "Changed setting hit Set CCD before continuing" <- FALSE ("Set CCD")
          }
        }
      }
      event "Cosmic Ray\nRemoval?", "ADC", "GAIN", "Time Between Acq. (ms)", "trigger Set CCD warning": Value Change {
        n181 = event-data() -> ()  [unwired: 1 in, 6 out]
        n182 = local write "Changed setting hit Set CCD before continuing"(TRUE ("trigger Set CCD warning")) -> ()
        n183 = local write "trigger Set CCD warning"(FALSE ("trigger Set CCD warning")) -> ()
      }
      event "Raster explanation": Value Change {
        n184 = event-data() -> ()  [unwired: 1 in, 6 out]
        n185 = flat-sequence {
          frame #0 {
            n186 = call "Display Message to User"() -> ()  [unwired: 10 in, 2 out]
          }
          frame #1 {
            n187 = local write "Raster explanation"(FALSE ("Raster explanation")) -> ()
          }
        }
      }
      event "Take Spectrum": Value Change {
        n188 = event-data() -> ()  [unwired: 1 in, 5 out]
        n189 = Bundle By Name(cluster=w376, "Raster Scan?"=FALSE ("Raster Scan.Raster Scan?")) -> (w375:refnum<class "Synapse CCD.lvclass">)
        n190 = flat-sequence {
          tunnel: [w402] -> w379
          tunnel: [w401] -> w378
          tunnel: [w398] -> w381
          tunnel: w377 -> [w396]
          tunnel: w375 -> [w393]
          tunnel: w379 -> [w405]
          tunnel: w378 -> [w407]
          tunnel: [w404] -> w380
          tunnel: [w406] -> w372
          tunnel: [w403] -> w388
          frame #0 {
            n191 = local read "Bin width (nm)\n(scan resolution)"() -> (w399:dbl[unit])
            n192 = call "Multi-Acq.vi"("error in"=w396, "Synapse CCD.lvclass In"=w393) -> ("error out"=w395:errorcluster, "Synapse CCD.lvclass Out"=w394:refnum<class "Synapse CCD.lvclass">)  [unwired: 7 in, 1 out]
            n193 = node(w399) -> (w400:dbl)
            n194 = call "Multi Data Processor.vi"("error in (no error)"=w395, "Step Size"=w400, "Synapse CCD.lvclass In"=w394) -> ("error out"=w401:errorcluster, "Processed Spectrum"=w398:cluster{"Ramp Pattern":dbl[], "X array":dbl[]}[], "Synapse CCD.lvclass Out"=w402:refnum<class "Synapse CCD.lvclass">, "Cosmic Ray Location(s)"=w397:string)  [unwired: 4 in, 1 out]
            n195 = local write "Cosmic Ray Locations"(w397) -> ()
          }
          frame #1 {
            n196 = local write "Take Spectrum"(FALSE ("Take Spectra")) -> ()
            n197 = call "Get Axis.vi"("error in (no error)"=w407, "Synapse CCD.lvclass in"=w405) -> ("error out"=w406:errorcluster, "Array of Wavelengths"=w403:dbl[], "Synapse CCD.lvclass out"=w404:refnum<class "Synapse CCD.lvclass">)  [unwired: 7 in]
          }
        }
        n198 = Index Array(array=w381, index=0) -> (element=w384:cluster{"Ramp Pattern":dbl[], "X array":dbl[]})
        n199 = Unbundle By Name(w384) -> ("X array"=w383:dbl[])
        n200 = Array Max & Min(array=w383) -> (max value=→"Max value of last snapshot":dbl)  [unwired: 3 out]
        n201 = Unbundle By Name(w380) -> ("Raw Data"=w392:i32[][])
        n202 = Index Array(array=w392) -> (element #1=w391:i32[], element #2=w387:i32[])  [unwired: 4 in]
        n203 = Bundle("Array of Wavelengths"=w388, "Raw Data"=w387) -> (w386:T10)  [unwired: 1 in]
        n204 = Bundle("Array of Wavelengths"=w388, "Raw Data"=w391) -> (w390:T10)  [unwired: 1 in]
        n205 = Build Array(w390, w386) -> (→"UnProcessed Spectra":T3)
        n206 = property on="Populate Fields with Member Data" class="Bool (strict)"(error in=w372, "Val(Sgnl)"=TRUE ("Value (Signaling)")) -> (error out=w371:errorcluster)  [unwired: 1 in, 1 out]
        "Spectrum" <- w381
      }
      event "Raster Scan": Value Change {
        n207 = event-data() -> ()  [unwired: 1 in, 5 out]
        n208 = local read "Raster Scan"() -> (w411:bool)
        n209 = case shown="True" w411 {
          tunnel: w414 -> [w415 w423]
          tunnel: [w415 w429] -> w409
          tunnel: w413 -> [w416 w425]
          tunnel: [w416 w428] -> w410
          tunnel: w412 -> [_ w424]
          frame False {
          }
          frame True {
            n210 = flat-sequence {
              tunnel: [w436] -> w422
              tunnel: [w435] -> w421
              tunnel: [w437] -> w420
              tunnel: [w432] -> w419
              tunnel: [w442] -> w418
              tunnel: [w441] -> w417
              tunnel: w425 -> [w433]
              tunnel: w424 -> [w442]
              tunnel: w423 -> [w441]
              tunnel: [w452] -> w427
              tunnel: [w451] -> w426
              tunnel: w422 -> [w450]
              tunnel: w421 -> [w449]
              tunnel: w420 -> [w448]
              tunnel: w419 -> [w447]
              tunnel: w418 -> [w446]
              tunnel: w417 -> [w445]
              tunnel: [w555] -> w428
              tunnel: [w556] -> w429
              tunnel: w427 -> [w556]
              tunnel: w426 -> [w555]
              frame #0 {
                w430 = FALSE ("Raster Scan.Warning: counts \nwent too high!")
                n211 = local read "Number of CCD bins to use each snapshot"() -> (w439:i32)
                n212 = local read "Bin width (nm)\n(scan resolution)"() -> (w440:dbl[unit])
                n213 = Bundle By Name(cluster=w433, "Raster Scan?"=TRUE ("Raster Scan.Raster Scan?"), "Warning: counts \nwent too high!"=w430) -> (w432:refnum<class "Synapse CCD.lvclass">)
                n214 = local read "Start"() -> (w434:dbl[unit])
                n215 = local read "End"() -> (w438:dbl[unit])
                n216 = local write "Warning: counts \nwent too high!"(w430) -> ()
                n217 = call "Raster Scan Init.vi"("Start"=w434, "Bins per scan"=w439, "Bin width (nm)"=w440, "End"=w438) -> ("Empty Data Array"=w437:cluster{dbl[unit], dbl[]}[], "Spec First Position"=w436:dbl[unit], "Number of CCD snapshots in scan"=w435:dbl)  [unwired: 4 in, 1 out]
              }
              frame #1 {
                n218 = while {
                  shift-right: [w494] -> w452
                  shift-left: w445 -> [w499]
                  tunnel: w446 -> [w500]
                  shift-right: [w455] -> w451
                  shift-left: w447 -> [w457]
                  shift-right: [w492] -> _
                  shift-left: w448 -> [w479]
                  shift-right: [w488] -> _
                  shift-left: 0.0 ("x") -> [w467]
                  tunnel: w450 -> [w465]
                  tunnel: w449 -> [w464]
                  tunnel: [w463] -> w444 mode=indexing
                  shift-right: [w454] -> _
                  shift-left: FALSE -> [w458]
                  i -> [w466]
                  stop <- w468 continue-if-true
                  # "If we have finished the captures for the raster scan,\nthe button will turn off and the loop will exit.\nIf someone pushes the button manually,\nthe loop will also exit."
                  n219 = local read "Bin width (nm)\n(scan resolution)"() -> (w493:dbl[unit])
                  n220 = Multiply(x=w493, y=w466) -> (x*y=w510:dbl[unit])
                  n221 = Unbundle By Name(w457) -> ("JYCCDLib.IJYCCDReqd"=w483:refnum<k7>, "JYMONOLib.IJYMonoReqd"=w484:refnum<k7>)
                  n222 = Increment(x=w467) -> (x+1=w488:dbl)
                  n223 = Add(x=w510, y=w465) -> (x+y=w498:dbl[unit])
                  n224 = Less Or Equal?(x=w488, y=w464) -> (x <= y?=w469:bool)
                  n225 = flat-sequence {
                    tunnel: w499 -> [w515]
                    tunnel: [w514] -> w509
                    tunnel: [w511] -> w508
                    tunnel: w500 -> [w513]
                    tunnel: [w512] -> w507
                    tunnel: w498 -> [w512]
                    tunnel: w484 -> [w511]
                    tunnel: w509 -> [w519]
                    tunnel: [w518] -> w506
                    tunnel: w508 -> [w516]
                    tunnel: [w516] -> w505
                    tunnel: [w520] -> w504
                    tunnel: w507 -> [w520]
                    tunnel: w506 -> [w523]
                    tunnel: [w523] -> w503
                    tunnel: w505 -> [w524]
                    tunnel: [w524] -> w502
                    tunnel: w504 -> [w522]
                    tunnel: [w522] -> w501
                    tunnel: w503 -> [w529]
                    tunnel: w502 -> [w530]
                    tunnel: w501 -> [w527]
                    tunnel: w483 -> [w525]
                    tunnel: [w535] -> w497
                    tunnel: [w532] -> w496
                    tunnel: [w526] -> w495
                    tunnel: w497 -> [w539]
                    tunnel: w496 -> [w540]
                    tunnel: w495 -> [w541]
                    tunnel: w457 -> [w549]
                    tunnel: [w545] -> w487
                    tunnel: [w544] -> w486
                    tunnel: [w537] -> w462
                    tunnel: [w552] -> w478
                    tunnel: [w553] -> w477
                    tunnel: w487 -> [w553]
                    tunnel: w486 -> [w552]
                    tunnel: [w551] -> w485
                    tunnel: [w550] -> w461
                    tunnel: w462 -> [w550]
                    frame #0 {
                      n226 = call "Move to Wavelength (TRIAX).vi"("error in (no error)"=w515, "Target wavelength"=w512, "VISA resource name"=w513) -> ("error out"=w514:errorcluster)  [unwired: 7 in, 1 out]
                    }
                    frame #1 {
                      n227 = property on="Populate Fields with Member Data" class="Bool (strict)"(error in=w519, "Val(Sgnl)"=TRUE ("Value (Signaling)")) -> (error out=w518:errorcluster)  [unwired: 1 in, 1 out]
                    }
                    frame #2 {
                      # "Pause so two \"sets\" \ndon't interfere"
                      n228 = Wait (ms)(milliseconds to wait=u32 100) -> ()  [unwired: 1 out]
                    }
                    frame #3 {
                      w536 = 13 items=["jyUndefined", "jypMonoLinearDispersion", "jypMonoBacklashAmount", "jypMonoStepsPerUnit", "jypMonoBaseUnits", "jypMonoBaseGrating", "jypMonoCurrentGrating", "jypMonoMaxLimit", "jypMonoMinLimit", "jypMonoTiltAngle", "jypMonoIncludedAngle", "jypMonoFocalLength", "jypMonoOrder", "jypMonoCurrentWavelength", "jypMonoMCDWavelengthDirection", "jypBandpassUnits", "jypSlitMaxLimit", "jypSlitMinLimit", "jypSlitBackLashAmount", "jypSlitBaseUnits", "jypSlitStepsPerUnit", "jypLaserLine", "jypTotalHardwarePropertiesPlusOne", "jypCurrentTurretPosition"] ("whichProperty")
                      # "This extra set is needed to keep \nthe Mono class \"in-the-know\""
                      n229 = node(w527) -> (w531:dbl)
                      n230 = call "JYMoveMono.vi"("error in (no error)"=w529, 10:w531, "JYMONOLib.IJYMonoReqd"=w530) -> ("error out"=w528:errorcluster)  [unwired: 8 in]
                      n231 = call "JYGetCurrentWL.vi"("error in (no error)"=w528, "JYMONOLib.IJYMonoReqd In"=w530) -> ("error out"=w533:errorcluster, "Current WL"=w534:dbl, "JYMONOLib.IJYMonoReqd Out"=w532:refnum<k7>)  [unwired: 6 in, 1 out]
                      n232 = invoke class="IJYCCDReqd" method="SetMonoProperty"(reference=w525, error in=w533, "whichProperty"=w536, "propVal"=w534) -> (reference out=w526:refnum<k7>, error out=w535:errorcluster)  [unwired: 1 in, 3 out]
                    }
                    frame #4 {
                      # "Take data"
                      n233 = Bundle By Name(cluster=w549, "JYCCDLib.IJYCCDReqd"=w541, "JYMONOLib.IJYMonoReqd"=w540) -> (w548:refnum<class "Synapse CCD.lvclass">)
                      n234 = local read "Bin width (nm)\n(scan resolution)"() -> (w543:dbl[unit])
                      n235 = call "Multi-Acq.vi"("error in"=w539, "Synapse CCD.lvclass In"=w548) -> ("error out"=w546:errorcluster, "max value"=w537:i32, "Synapse CCD.lvclass Out"=w547:refnum<class "Synapse CCD.lvclass">)  [unwired: 7 in]
                      n236 = node(w543) -> (w542:dbl)
                      n237 = call "Multi Data Processor.vi"("error in (no error)"=w546, "Step Size"=w542, "Synapse CCD.lvclass In"=w547) -> ("error out"=w545:errorcluster, "Synapse CCD.lvclass Out"=w544:refnum<class "Synapse CCD.lvclass">, "Cosmic Ray Location(s)"=w538:string)  [unwired: 4 in, 2 out]
                      n238 = local write "Cosmic Ray Locations"(w538) -> ()
                    }
                    frame #5 {
                      n239 = local read "Raster Scan"() -> (w551:bool)
                    }
                  }
                  n240 = local read "Number of CCD bins to use each snapshot"() -> (w482:i32)
                  n241 = local read "Bin width (nm)\n(scan resolution)"() -> (w481:dbl[unit])
                  n242 = local read "Start"() -> (w480:dbl[unit])
                  n243 = local read "End"() -> (w491:dbl[unit])
                  n244 = Unbundle By Name(w478) -> ("Processed Data"=w490:dbl[])
                  n245 = Unbundle By Name(w478) -> ()  [unwired: 1 out]
                  n246 = Unbundle By Name(w457) -> ()  [unwired: 1 out]
                  n247 = call "Get Axis.vi"("error in (no error)"=w477, "Synapse CCD.lvclass in"=w478) -> ("error out"=w494:errorcluster, "Array of Wavelengths"=w476:dbl[], "Synapse CCD.lvclass out"=w475:refnum<class "Synapse CCD.lvclass">)  [unwired: 7 in]
                  n248 = Bundle("Array of Wavelengths"=w476, "Processed Data"=w490) -> (w489:T11)  [unwired: 1 in]
                  n249 = call "Insert data into array.vi"("current snapshot number"=w467, "End wavelength of raster scan"=w491, "To Append"=w489, "Start wavelength of raster scan"=w480, "Bins per scan"=w482, "Bin width (nm)"=w481, "Main data array for raster scan, before this this snapshot"=w479) -> ("new version of Emma and John Data Array for current snapshot"=w463:i32[], "Main data array for raster scan,\nas modified after this snapshot"=w492:cluster{dbl[unit], dbl[]}[])  [unwired: 3 in]
                  n250 = local write "Max value of last snapshot"(w461) -> ()
                  n251 = call "Process Raster Data.vi"("Input Array"=w492) -> ("Avg Counts"=w472:dbl[], "Raw Counts"=w474:dbl[][], "Wavelengths"=w473:dbl[])  [unwired: 8 in]
                  n252 = Bundle By Name(cluster=w475, "Processed Data"=w472, "Raw Data"=w474, "Array of Wavelengths"=w473) -> (w456:refnum<class "Synapse CCD.lvclass">)
                  n253 = And(x=w485, y=w469) -> (x .and. y?=w468:bool)
                  n254 = Bundle("Wavelengths"=w473, "Avg Counts"=w472) -> (w471:cluster{"Wavelengths":dbl[], "Avg Counts":dbl[]})  [unwired: 1 in]
                  n255 = Equal?(x=w461, y=65535) -> (x = y?=w459:bool)
                  n256 = Build Array(w471) -> (w470:T12)
                  n257 = Or(x=w458, y=w459) -> (x .or. y?=w454:bool)
                  n258 = local write "Warning: counts \nwent too high!"(w454) -> ()
                  n259 = local write "Spectrum"(w470) -> ()
                  n260 = Bundle By Name(cluster=w456, "Warning: counts \nwent too high!"=w454) -> (w455:refnum<class "Synapse CCD.lvclass">)
                  "Current snapshot" <- w466
                }
                "new version of 2D Emma and John Array" <- w444
              }
              frame #2 {
                n261 = local write "Raster Scan"(FALSE ("Take Spectra")) -> ()
              }
            }
          }
        }
      }
      event "Go to start\nof raster scan": Value Change {
        n262 = event-data() -> ()  [unwired: 1 in, 6 out]
        n263 = flat-sequence {
          frame #0 {
            n264 = Wait (ms)(milliseconds to wait=u32 100) -> ()  [unwired: 1 out]
            n265 = local read "Start"() -> (w560:dbl[unit])
            n266 = property on="Center Wavelength" class="DigNum (strict)"("Val(Sgnl)"=w560) -> ()  [unwired: 2 in, 2 out]
          }
          frame #1 {
            n267 = local write "Go to start\nof raster scan"(FALSE ("Go to start of raster scan")) -> ()
          }
        }
      }
      event "Start", "Bin width (nm)\n(scan resolution)", "Number of CCD bins to use each snapshot", "Bin width (pixels)", "End", "Resolution\n(nm/pixel)": Value Change {
        n268 = event-data() -> ()  [unwired: 1 in, 6 out]
        n269 = flat-sequence {
          tunnel: [w602] -> w565
          frame #0 {
            # "Calculate bin width in nm and Total possible CCD bins"
            n270 = local read "Resolution\n(nm/pixel)"() -> (w606:dbl[unit])
            n271 = local read "Bin width (pixels)"() -> (w605:i32)
            n272 = Multiply(x=w606, y=w605) -> (x*y=w602:dbl[unit])
            n273 = Divide(x=1024.0, y=w605) -> (x/y=w604:dbl)
            n274 = local write "Total possible CCD bins"(w604) -> ()
            n275 = local write "Bin width (nm)\n(scan resolution)"(w602) -> ()
          }
        }
        n276 = flat-sequence {
          tunnel: w565 -> [w570]
          tunnel: w563 -> [w595]
          tunnel: [w594] -> w562
          frame #0 {
            # "Basic logic for this calculation (doesn't take into account time for spectrometer to move):\nexpected time = number of snapshots x time for a snapshot\ntime for a snapshot = number of aquisitions per snapshot x (integration time + shutter open/close time)\nnumber of aquisitions per snapshot = number to average, plus one extra if dark subtract"
            n277 = flat-sequence {
              tunnel: [w586] -> w569
              frame #0 {
                w592 = u32 1 ("upper limit")
                n278 = local read "# to Average"() -> (w591:u32)
                n279 = Less?(x=w591, y=w592) -> (x < y?=w593:bool)
                n280 = local read "Dark Subtract?"() -> (w590:bool)
                n281 = Select "# to average: if it's less \nthan 1, then set it equal to 1"(t=w592, s=w593, f=w591) -> (s? t:f=w583:u32)
                n282 = local read "Averaging?"() -> (w585:bool)
                n283 = Select "if dark subtract, need\nto do one addl scan"(t=1, s=w590, f=0) -> (s? t:f=w587:i32)
                n284 = Select "if not averaging, then just 1"(t=w583, s=w585, f=1) -> (s? t:f=w582:u32)
                n285 = Add "number of \naquisitions \nper snapshot"(x=w582, y=w587) -> (x+y=w586:u32)
              }
            }
            n286 = flat-sequence {
              tunnel: w570 -> [w573]
              tunnel: [w572] -> w568
              frame #0 {
                n287 = local read "Number of CCD bins to use each snapshot"() -> (w574:i32)
                n288 = local read "End"() -> (w576:dbl[unit])
                n289 = local read "Start"() -> (w575:dbl[unit])
                n290 = call "calculate number of data points and number of snapshots.vi"("Number of CCD bins to use each snapshot"=w574, "Bin width (nm)\n(scan resolution)"=w573, "Start"=w575, "End"=w576) -> ("Number of snapshots required for scan"=w572:dbl, "Number of data points in scan"=→"Number of data \npoints required":dbl)  [unwired: 6 in]
                "Number of snap-\nshots required" <- w572
              }
            }
            n291 = flat-sequence {
              tunnel: w569 -> [w580]
              tunnel: [w577] -> w566
              frame #0 {
                w581 = dbl[unit] 0.125  # about how long to open and close shutter
                n292 = local read "Integration time"() -> (w579:dbl[unit])
                n293 = Add "time for an acquisition"(x=w579, y=w581) -> (x+y=w578:dbl[unit])
                n294 = Multiply "time for a snapshot"(x=w580, y=w578) -> (x*y=w577:dbl[unit])
              }
            }
            n295 = Multiply(x=w568, y=w566) -> (x*y=→"Expected time":dbl[unit])
          }
          frame #1 {
            n296 = local read "Start"() -> (w596:dbl[unit])
            n297 = local read "End"() -> (w597:dbl[unit])
            n298 = local read "Bin width (pixels)"() -> (w598:i32)
            n299 = local read "Bin width (nm)\n(scan resolution)"() -> (w599:dbl[unit])
            n300 = local read "Number of CCD bins to use each snapshot"() -> (w600:i32)
            n301 = local read "Total possible CCD bins"() -> (w601:dbl)
            n302 = Bundle By Name(cluster=w595, "Start"=w596, "End"=w597, "Bin width (pixels)"=w598, "Bin width (nm)\n(scan resolution)"=w599, "Number of CCD bins to use each snapshot"=w600, "Total possible CCD bins"=w601) -> (w594:refnum<class "Synapse CCD.lvclass">)
          }
        }
      }
      event "Integration time", "Averaging?", "# to Average", "Dark Subtract?": Value Change {
        n303 = event-data() -> ()  [unwired: 1 in, 6 out]
        n304 = flat-sequence {
          tunnel: [w648] -> w610
          frame #0 {
            # "Calculate bin width in nm and Total possible CCD bins"
            n305 = local read "Resolution\n(nm/pixel)"() -> (w652:dbl[unit])
            n306 = local read "Bin width (pixels)"() -> (w651:i32)
            n307 = Multiply(x=w652, y=w651) -> (x*y=w648:dbl[unit])
            n308 = Divide(x=1024.0, y=w651) -> (x/y=w650:dbl)
            n309 = local write "Total possible CCD bins"(w650) -> ()
            n310 = local write "Bin width (nm)\n(scan resolution)"(w648) -> ()
          }
        }
        n311 = flat-sequence {
          tunnel: w610 -> [w615]
          tunnel: w608 -> [w641]
          tunnel: [w640] -> w607
          frame #0 {
            # "Basic logic for this calculation (doesn't take into account time for spectrometer to move):\nexpected time = number of snapshots x time for a snapshot\ntime for a snapshot = number of aquisitions per snapshot x (integration time + shutter open/close time)\nnumber of aquisitions per snapshot = number to average, plus one extra if dark subtract"
            n312 = flat-sequence {
              tunnel: [w631] -> w614
              frame #0 {
                w637 = u32 1 ("upper limit")
                n313 = local read "# to Average"() -> (w636:u32)
                n314 = Less?(x=w636, y=w637) -> (x < y?=w638:bool)
                n315 = local read "Dark Subtract?"() -> (w635:bool)
                n316 = Select "# to average: if it's less \nthan 1, then set it equal to 1"(t=w637, s=w638, f=w636) -> (s? t:f=w628:u32)
                n317 = local read "Averaging?"() -> (w630:bool)
                n318 = Select "if dark subtract, need\nto do one addl scan"(t=1, s=w635, f=0) -> (s? t:f=w632:i32)
                n319 = Select "if not averaging, then just 1"(t=w628, s=w630, f=1) -> (s? t:f=w627:u32)
                n320 = Add "number of \naquisitions \nper snapshot"(x=w627, y=w632) -> (x+y=w631:u32)
              }
            }
            n321 = flat-sequence {
              tunnel: w615 -> [w618]
              tunnel: [w616] -> w613
              frame #0 {
                n322 = local read "Number of CCD bins to use each snapshot"() -> (w619:i32)
                n323 = local read "End"() -> (w621:dbl[unit])
                n324 = local read "Start"() -> (w620:dbl[unit])
                n325 = call "calculate number of data points and number of snapshots.vi"("Number of CCD bins to use each snapshot"=w619, "Bin width (nm)\n(scan resolution)"=w618, "Start"=w620, "End"=w621) -> ("Number of snapshots required for scan"=w616:dbl, "Number of data points in scan"=w617:dbl)  [unwired: 6 in]
                n326 = local write "Number of data \npoints required"(w617) -> ()
                n327 = local write "Number of snap-\nshots required"(w616) -> ()
              }
            }
            n328 = flat-sequence {
              tunnel: w614 -> [w625]
              tunnel: [w622] -> w612
              frame #0 {
                w626 = dbl[unit] 0.125  # about how long to open and close shutter
                n329 = local read "Integration time"() -> (w624:dbl[unit])
                n330 = Add "time for an acquisition"(x=w624, y=w626) -> (x+y=w623:dbl[unit])
                n331 = Multiply "time for a snapshot"(x=w625, y=w623) -> (x*y=w622:dbl[unit])
              }
            }
            n332 = Multiply(x=w613, y=w612) -> (x*y=w611:dbl[unit])
            n333 = local write "Expected time"(w611) -> ()
          }
          frame #1 {
            n334 = local read "Start"() -> (w642:dbl[unit])
            n335 = local read "End"() -> (w643:dbl[unit])
            n336 = local read "Bin width (pixels)"() -> (w644:i32)
            n337 = local read "Bin width (nm)\n(scan resolution)"() -> (w645:dbl[unit])
            n338 = local read "Number of CCD bins to use each snapshot"() -> (w646:i32)
            n339 = local read "Total possible CCD bins"() -> (w647:dbl)
            n340 = property on="trigger Set CCD warning" class="Bool (strict)"("Val(Sgnl)"=TRUE ("trigger Set CCD warning")) -> ()  [unwired: 2 in, 2 out]
            n341 = Bundle By Name(cluster=w641, "Start"=w642, "End"=w643, "Bin width (pixels)"=w644, "Bin width (nm)\n(scan resolution)"=w645, "Number of CCD bins to use each snapshot"=w646, "Total possible CCD bins"=w647) -> (w640:refnum<class "Synapse CCD.lvclass">)
          }
        }
      }
      event "Repeat Capture": Value Change {
        n342 = event-data() -> ()  [unwired: 1 in, 5 out]
        n343 = Bundle By Name(cluster=w658, "Raster Scan?"=FALSE ("Raster Scan.Raster Scan?")) -> (w657:refnum<class "Synapse CCD.lvclass">)
        n344 = local read "Repeat Capture"() -> (w660:bool)
        n345 = case shown="True" w660 {
          tunnel: w661 -> [w663 w667]
          tunnel: [w663 w666] -> w654
          tunnel: w657 -> [w662 w665]
          tunnel: [w662 w664] -> w659
          frame False {
          }
          frame True {
            n346 = while {
              tunnel: w667 -> [w693]
              tunnel: [w692] -> w666
              tunnel: w665 -> [w691]
              tunnel: [w673] -> w664
              stop <- w674 continue-if-true
              n347 = flat-sequence {
                tunnel: w693 -> [w700]
                tunnel: w691 -> [w703]
                tunnel: [w701] -> w682
                tunnel: [w698] -> w680
                tunnel: [w695] -> w683
                tunnel: [w694] -> w668
                tunnel: w682 -> [w707]
                tunnel: [w707] -> w681
                tunnel: w680 -> [w706]
                tunnel: [w706] -> w679
                tunnel: "Repeat pause (ms)" -> [w705]
                tunnel: w668 -> [w704]
                tunnel: w681 -> [w710]
                tunnel: w679 -> [w712]
                tunnel: [w709] -> w677
                tunnel: [w711] -> w676
                tunnel: [w708] -> w675
                tunnel: [w714] -> w689
                tunnel: [w715] -> w692
                tunnel: [w716] -> w673
                tunnel: w677 -> [w716]
                tunnel: w676 -> [w715]
                tunnel: w675 -> [w714]
                tunnel: [w713] -> w674
                frame #0 {
                  n348 = local read "Bin width (nm)\n(scan resolution)"() -> (w697:dbl[unit])
                  n349 = call "Multi-Acq.vi"("error in"=w700, "Synapse CCD.lvclass In"=w703) -> ("error out"=w699:errorcluster, "Synapse CCD.lvclass Out"=w702:refnum<class "Synapse CCD.lvclass">)  [unwired: 7 in, 1 out]
                  n350 = node(w697) -> (w696:dbl)
                  n351 = call "Multi Data Processor.vi"("error in (no error)"=w699, "Step Size"=w696, "Synapse CCD.lvclass In"=w702) -> ("error out"=w698:errorcluster, "Processed Spectrum"=w695:cluster{"Ramp Pattern":dbl[], "X array":dbl[]}[], "Synapse CCD.lvclass Out"=w701:refnum<class "Synapse CCD.lvclass">, "Cosmic Ray Location(s)"=w694:string)  [unwired: 4 in, 1 out]
                }
                frame #1 {
                  n352 = local write "Cosmic Ray Locations"(w704) -> ()
                  n353 = Wait (ms)(milliseconds to wait=w705) -> ()  [unwired: 1 out]
                }
                frame #2 {
                  n354 = call "Get Axis.vi"("error in (no error)"=w712, "Synapse CCD.lvclass in"=w710) -> ("error out"=w711:errorcluster, "Array of Wavelengths"=w708:dbl[], "Synapse CCD.lvclass out"=w709:refnum<class "Synapse CCD.lvclass">)  [unwired: 7 in]
                }
                frame #3 {
                  n355 = local read "Repeat Capture"() -> (w713:bool)
                }
              }
              n356 = Index Array(array=w683, index=0) -> (element=w685:cluster{"Ramp Pattern":dbl[], "X array":dbl[]})
              n357 = local write "Spectrum"(w683) -> ()
              n358 = Unbundle By Name(w685) -> ("X array"=w684:dbl[])
              n359 = Array Max & Min(array=w684) -> (max value=w687:dbl)  [unwired: 3 out]
              n360 = local write "Max value of last snapshot"(w687) -> ()
              n361 = Unbundle By Name(w673) -> ("Raw Data"=w672:i32[][])
              n362 = Index Array(array=w672) -> (element #1=w690:i32[], element #2=w688:i32[])  [unwired: 4 in]
              n363 = Bundle("Array of Wavelengths"=w689, "Raw Data"=w690) -> (w671:T10)  [unwired: 1 in]
              n364 = Bundle("Array of Wavelengths"=w689, "Raw Data"=w688) -> (w670:T10)  [unwired: 1 in]
              n365 = Build Array(w671, w670) -> (w669:T3)
              n366 = local write "UnProcessed Spectra"(w669) -> ()
            }
          }
        }
        n367 = property on="Populate Fields with Member Data" class="Bool (strict)"(error in=w654, "Val(Sgnl)"=TRUE ("Value (Signaling)")) -> (error out=w653:errorcluster)  [unwired: 1 in, 1 out]
      }
      event "image mode": Value Change {
        n368 = event-data() -> ()  [unwired: 1 in, 6 out]
        n369 = vi-ref "Image mode.vi"() -> (w718:refnum<vi>)
        n370 = call "Application Launcher.vi"("Toggle?"="image mode", "VI reference"=w718) -> ()  [unwired: 1 in, 9 out]
      }
      event "Export\nPlot": Value Change {
        n371 = event-data() -> ()  [unwired: 1 in, 5 out]
        n372 = flat-sequence {
          tunnel: w723 -> [w732]
          tunnel: w724 -> [w735]
          tunnel: [w731] -> w722
          tunnel: [w733] -> w720
          tunnel: w720 -> [w737]
          tunnel: [w737] -> w719
          tunnel: [w738] -> w721
          tunnel: w719 -> [w739]
          frame #0 {
            n373 = local read "Status"() -> (w728:string)
            n374 = Concatenate Strings("Comments", "\r", "==========" ("string"), "\r", w728) -> (w729:string)
            n375 = call "SaveData.vi"("error in (no error)"=w732, "Comments"=w729, "File Name"="File Name", "Synapse CCD.lvclass In"=w735) -> ("error out"=w733:errorcluster, "Synapse CCD.lvclass Out"=w731:refnum<class "Synapse CCD.lvclass">)  [unwired: 6 in]
          }
          frame #1 {
            n376 = Wait (ms)(milliseconds to wait=u32 100) -> ()  [unwired: 1 out]
          }
          frame #2 {
            n377 = call <vilib>:"Simple Error Handler.vi"("error in (no error)"=w739) -> ("error out"=w738:errorcluster)  [unwired: 4 in, 4 out]
            n378 = local write "Export\nPlot"(FALSE) -> ()
          }
        }
      }
      event "stop": Value Change {
        n379 = event-data() -> ()  [unwired: 1 in, 5 out]
      }
    }
  }
  n380 = call-dynamic "_Destroy.vi"("error in (no error)"=w3, "Synapse CCD in"=w1) -> ("error out"=→"error out":errorcluster)  [unwired: 9 in]
  n381 = Unbundle By Name(w1) -> ()  [unwired: 11 out]
